vi "Write Multiline.vi"(8 "error in (no error)":errorcluster, 10 "Multiline":bool, 11 "JSON Serializer in":refnum<class "JSON Serializer.lvclass">) -> (0 "error out":errorcluster, 3 "JSON Serializer out":refnum<class "JSON Serializer.lvclass">)   [LabVIEW 2019, in "JKI JSON Serialization.lvlib" / "JSON Serializer.lvclass"]
doc: "Specifies if JSON string generated will be a compact single-line string (false) or pretty-printed multi-line string (true)?\n\nJKI JSON 1.1.10.37\nTomi Maila - JKI\nCopyright (c) 2017, JKI"
uses:
  JSON Serializer.lvclass
  JSON Serializer.lvclass/JSON Serializer.ctl
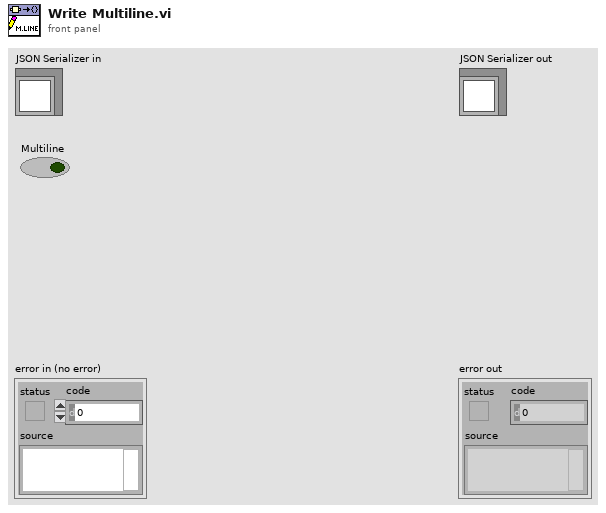
[diagram p1: front panel]
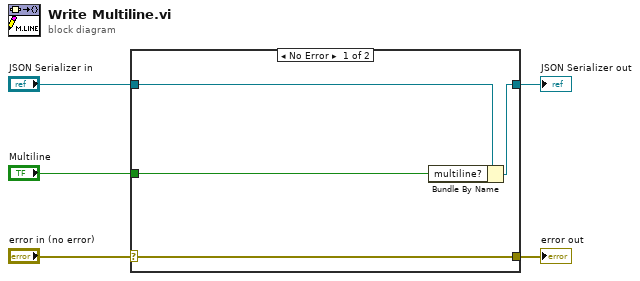
[diagram p0: block diagram]
diagram:
  n1 = case shown="No Error" "error in (no error)" {
    selector: "error in (no error)" -> [w9 w10]
    tunnel: [w9 w10] -> w4
    tunnel: [w7 w11] -> w2
    tunnel: "JSON Serializer in" -> [w8 w11]
    tunnel: "Multiline" -> [w6 _]
    frame No Error {
      n2 = Bundle By Name(cluster=w8, "multiline?"=w6) -> (w7:refnum<class "JSON Serializer.lvclass">)
    }
    frame Error {
    }
  }
  "error out" <- w4
  "JSON Serializer out" <- w2
